vi "Parse Parameter - Body.vi"(8 "error in (no error)":errorcluster, 11 "Body":string) -> (0 "error out":errorcluster, 3 "Body Parameters":T1[](array[typedef]))   [LabVIEW 2011, in "i3-oauth.lvlib"]
uses:
  i3-oauth.lvlib
  Controls/key-value-pairs.ctl
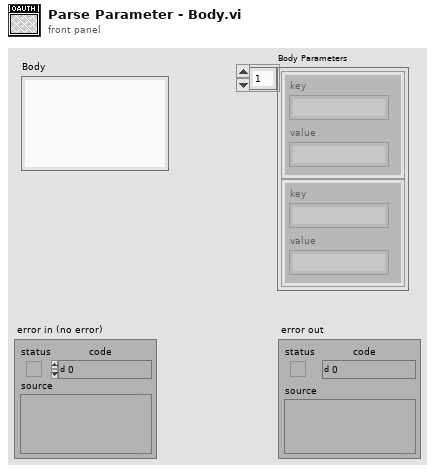
[diagram p1: front panel]
types:
  T1 = typedef "i3-oauth.lvlib/key-value-pairs.ctl" = cluster{"key":string, "value":string}
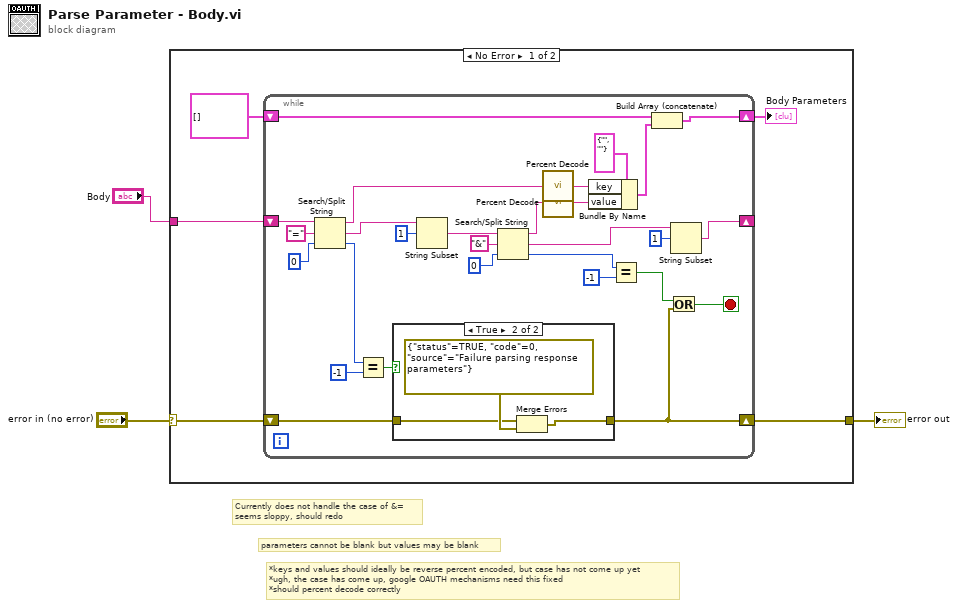
[diagram p0: block diagram]
diagram:
  # "*keys and values should ideally be reverse percent encoded, but case has not come up yet\n*ugh, the case has come up, google OAUTH mechanisms need this fixed\n*should percent decode correctly"
  # "parameters cannot be blank but values may be blank"
  # "Currently does not handle the case of &=\nseems sloppy, should redo"
  n1 = case shown="No Error" "error in (no error)" {
    selector: "error in (no error)" -> [w5 w41]
    tunnel: "Body" -> [w8 _]
    tunnel: [w4 w41] -> w1
    frame No Error {
      n2 = while {
        shift-right: [w29] -> w6
        shift-left: T1[] [] ("Body Parameters") -> [w31]
        shift-right: [w13] -> w4
        shift-left: w5 -> [w14]
        shift-right: [w17] -> _
        shift-left: w8 -> [w35]
        stop <- w24 stop-if-true
        n3 = Search/Split String(string=w35, search string/char (-)="=", offset (0)=0) -> (substring before match=w9:string, match + rest of string=w23:string, offset of match=w26:i32)
        n4 = Equal?(x=w26, y=-1) -> (x = y?=w15:bool)
        n5 = case shown="True" w15 {
          tunnel: w14 -> [w37 w39]
          tunnel: [w37 w38] -> w13
          frame False {
          }
          frame True {
            n6 = Merge Errors(w39, errorcluster {"status"=TRUE, "code"=0, "source"="Failure parsing response parameters"} ("error in (no error)")) -> (w38:errorcluster)
          }
        }
        n7 = String Subset(string=w23, offset (0)=1) -> (substring=w22:string)  [unwired: 1 in]
        n8 = Search/Split String(string=w22, search string/char (-)="&", offset (0)=0) -> (substring before match=w11:string, match + rest of string=w16:string, offset of match=w28:i32)
        n9 = call "Percent Decode.vi"("escaped string in"=w9) -> ("unescaped string out"=w10:string)
        n10 = call "Percent Decode.vi"("escaped string in"=w11) -> ("unescaped string out"=w12:string)
        n11 = Bundle By Name(cluster=T1 {"key"="", "value"=""} ("Key Value Pair"), "key"=w10, "value"=w12) -> (w30:T1)
        n12 = Equal?(x=w28, y=-1) -> (x = y?=w25:bool)
        n13 = Build Array (concatenate)(w31, w30) -> (w29:T1[])
        n14 = Or(x=w25, y=w13) -> (x .or. y?=w24:bool)
        n15 = String Subset(string=w16, offset (0)=1) -> (substring=w17:string)  [unwired: 1 in]
      }
      "Body Parameters" <- w6
    }
    frame Error {
    }
  }
  "error out" <- w1
